vi "VITree.vi"() -> ()   [LabVIEW 2009]
uses:
  <userlib>/_OpenG.lib/array/array.llb/Conditional Auto-Indexing Tunnel (Path)__ogtk.vi
panel:
  in  "Level":i32=2
  out "Arbre":string(tree)
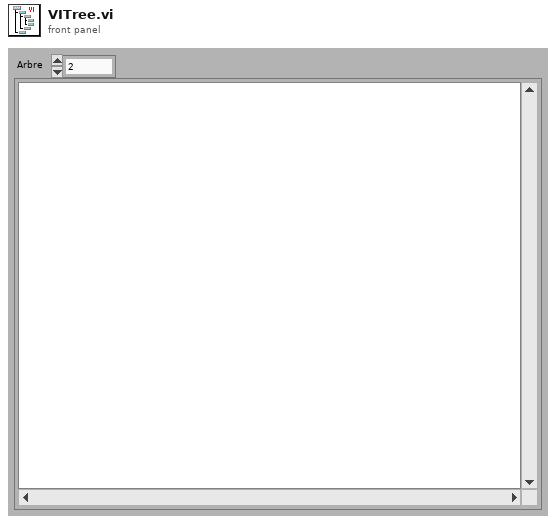
[diagram p1: front panel]
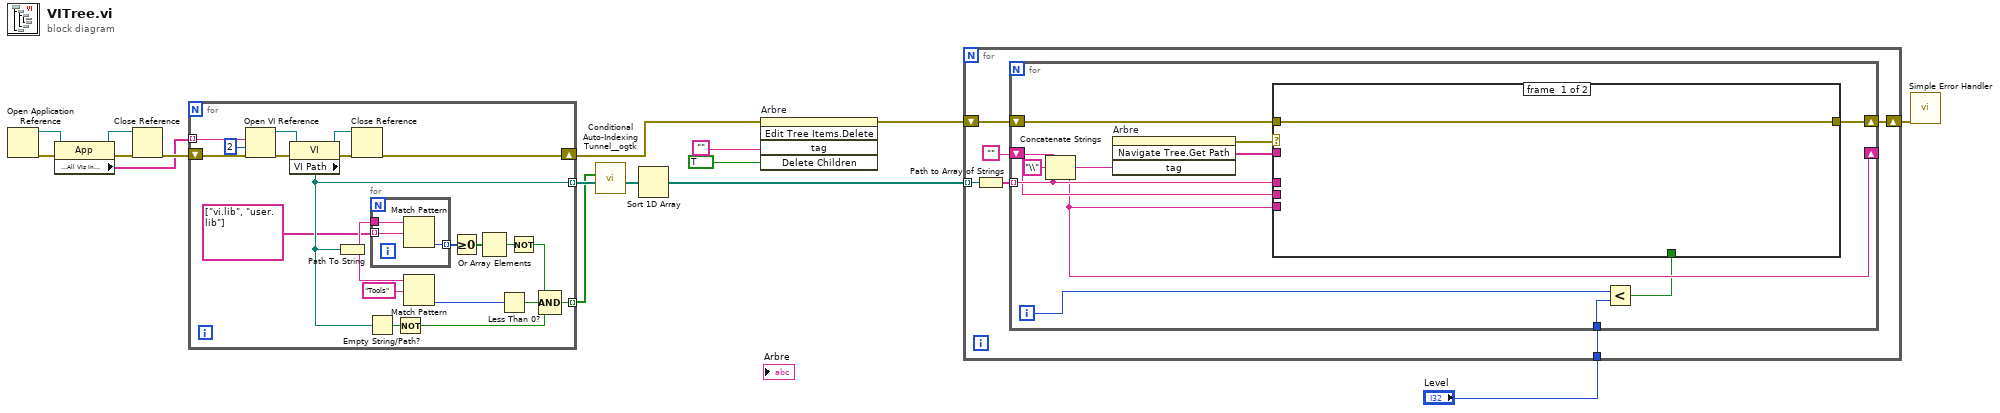
[diagram p0: block diagram]
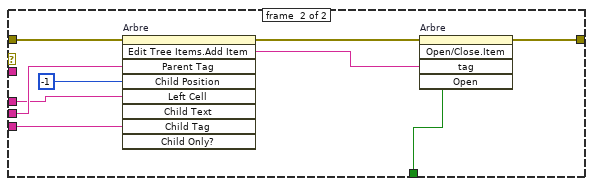
[diagram p2: hidden frame]
diagram:
  n1 = Open Application Reference() -> (0:w16:errorcluster, 3:w15:refnum<vi>)  [unwired: 1 in, 3 out]
  n2 = property class="App"(reference=w15, error in=w16) -> (reference out=w13:refnum<vi>, error out=w14:errorcluster, "Application:All VIs In Memory"=w11:string[])
  n3 = Close Reference(reference=w13, error in (no error)=w14) -> (error out=w12:errorcluster)
  n4 = for {
    shift-right: [w31] -> w9
    shift-left: w12 -> [w37]
    tunnel: w11 -> [w36] mode=indexing
    tunnel: [w25] -> w2 mode=indexing
    tunnel: [w24] -> w4 mode=indexing
    n5 = Open VI Reference(vi path=w36, options=2, error in (no error)=w37) -> (vi reference=w34:refnum<vi>, error out=w35:errorcluster)  [unwired: 3 out]
    n6 = property class="VI"(reference=w34, error in=w35) -> (reference out=w32:refnum<vi>, error out=w33:errorcluster, "VI Path"=w24:path)
    n7 = Path To String(path=w24) -> (string=w20:string)
    n8 = Close Reference(reference=w32, error in (no error)=w33) -> (error out=w31:errorcluster)
    n9 = Empty String/Path?(string/path=w24) -> (empty?=w23:bool)
    n10 = for {
      tunnel: [w40] -> w30 mode=indexing
      tunnel: w20 -> [w39]
      tunnel: string[] ["vi.lib", "user.lib"] -> [w38] mode=indexing
      n11 = Match Pattern(string=w39, regular expression=w38) -> (offset past match=w40:i32)  [unwired: 4 out]
    }
    n12 = Not(x=w23) -> (.not. x?=w22:bool)
    n13 = Match Pattern(string=w20, regular expression="Tools" ("expression régulière")) -> (offset past match=w29:i32)  [unwired: 4 out]
    n14 = Greater Or Equal To 0?(x=w30) -> (x >= 0?=w26:bool[])
    n15 = Or Array Elements(Boolean array=w26) -> (logical OR=w18:bool)
    n16 = Less Than 0?(x=w29) -> (x < 0?=w27:bool)
    n17 = Not(x=w18) -> (.not. x?=w17:bool)
    n18 = Compound Arithmetic op=AND(w17, w27, w22) -> (w25:bool)
  }
  n19 = call-poly <userlib>:"Conditional Auto-Indexing Tunnel__ogtk.vi"("Array in"=w4, "Elements to keep"=w2) -> ("Filtered Array out"=w3:path[])  [unwired: 5 out]
  n20 = Sort 1D Array(array=w3) -> (sorted array=w8:path[])
  n21 = invoke on="Arbre" class="CommandeArbre (strict)" method="Edit Tree Items.Delete"(error in=w9, "tag"="", "Delete Children"=TRUE ("Supprimer les fils")) -> (error out=w7:errorcluster)  [unwired: 2 in, 4 out]
  n22 = for {
    tunnel: w8 -> [w46] mode=indexing
    shift-right: [w43] -> w6
    shift-left: w7 -> [w45]
    tunnel: "Level" -> [w41]
    n23 = Path to Array of Strings(0:w46) -> (2:w44:string[])  [unwired: 1 out]
    n24 = for {
      shift-right: [w54] -> w43
      shift-left: w45 -> [w55]
      tunnel: w44 -> [w56] mode=indexing
      shift-right: [w50] -> _
      shift-left: "" -> [w51]
      tunnel: w41 -> [w49]
      i -> [w48]
      n25 = Concatenate Strings(w51, "\\" ("chaîne"), w56) -> (w50:string)
      n26 = invoke on="Arbre" class="CommandeArbre (strict)" method="Navigate Tree.Get Path"("tag"=w50) -> (error out=w53:errorcluster, "Navigate Tree:Get Path"=w52:string[])  [unwired: 3 in, 2 out]
      n27 = Less?(x=w48, y=w49) -> (x < y?=w47:bool)
      n28 = case shown="Error" w53 {
        tunnel: w56 -> [_ w63]
        tunnel: w55 -> [w58 w67]
        tunnel: [w58 w61] -> w54
        tunnel: w52 -> [_ _]
        tunnel: w51 -> [_ w65]
        tunnel: w50 -> [_ w64]
        tunnel: w47 -> [_ w59]
        frame #0 {
        }
        frame #1 {
          n29 = invoke on="Arbre" class="CommandeArbre (strict)" method="Edit Tree Items.Add Item"(error in=w67, "Parent Tag"=w65, "Child Position"=-1 ("Position du fils"), "Left Cell"=w63, "Child Tag"=w64) -> (error out=w62:errorcluster, "Edit Tree Items:Add Item"=w60:string)  [unwired: 4 in, 7 out]
          n30 = invoke on="Arbre" class="CommandeArbre (strict)" method="Open/Close.Item"(error in=w62, "tag"=w60, "Open"=w59) -> (error out=w61:errorcluster)  [unwired: 2 in, 4 out]
        }
      }
    }
  }
  n31 = call <vilib>:"Simple Error Handler.vi"("error in (no error)"=w6) -> ()  [unwired: 1 in, 8 out]
